vi "initUI.vi"(8 "Error In":errorcluster, 11 "UI Elements Cluster":T1) -> (0 "Error Out":errorcluster)   [LabVIEW 2018]
uses:
  controls/mainAppElementsCluster.ctl
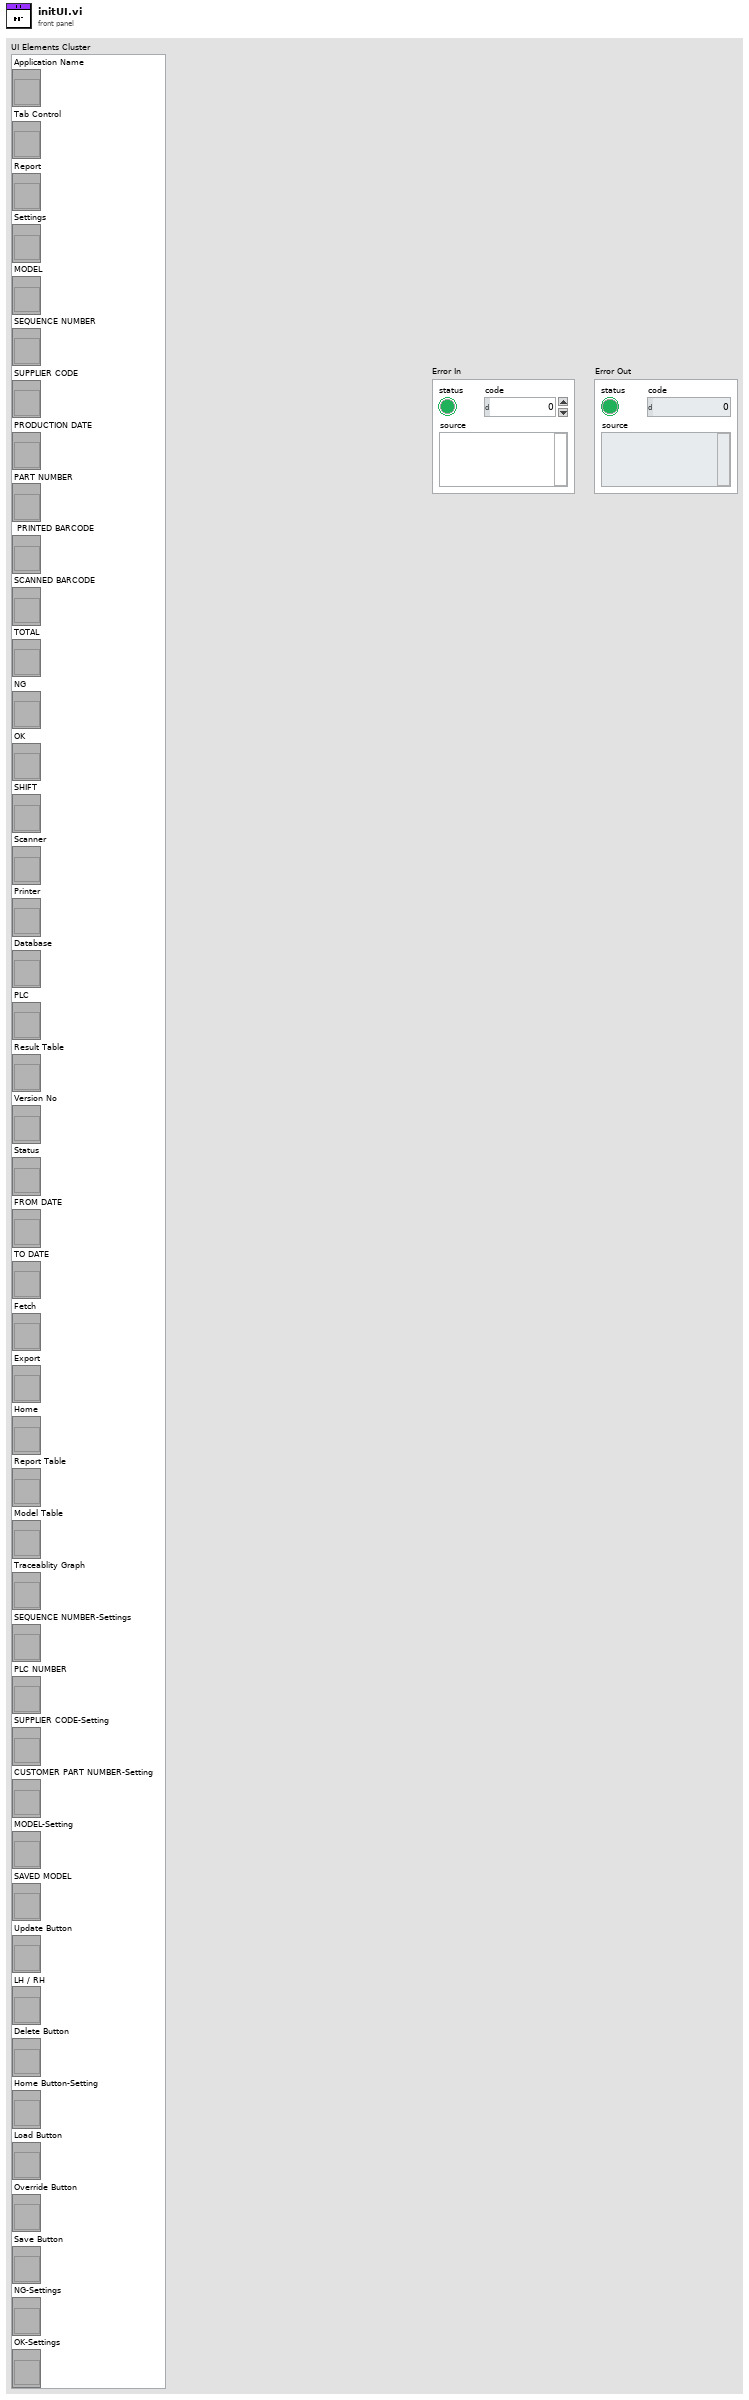
[diagram p1: front panel]
types:
  T1 = typedef "mainAppElementsCluster.ctl" = cluster{"Application Name":refnum<vi>, "Tab Control":refnum<vi>, "Status":refnum<vi>, "Version No":refnum<vi>, "Result Table":refnum<vi>, "PLC":refnum<vi>, "Database":refnum<vi>, "Printer":refnum<vi>, "Scanner":refnum<vi>, "SHIFT":refnum<vi>, "OK":refnum<vi>, "NG":refnum<vi>, "TOTAL":refnum<vi>, "SCANNED BARCODE":refnum<vi>, " PRINTED BARCODE":refnum<vi>, "PART NUMBER":refnum<vi>, "PRODUCTION DATE":refnum<vi>, "SUPPLIER CODE":refnum<vi>, "SEQUENCE NUMBER":refnum<vi>, "MODEL":refnum<vi>, "Settings":refnum<vi>, "Report":refnum<vi>, "Report Table":refnum<vi>, "Home":refnum<vi>, "Export":refnum<vi>, "Fetch":refnum<vi>, "TO DATE":refnum<vi>, "FROM DATE":refnum<vi>, "Model Table":refnum<vi>, "Traceablity Graph":refnum<vi>, "Override Button":refnum<vi>, "Load Button":refnum<vi>, "Home Button-Setting":refnum<vi>, "Delete Button":refnum<vi>, "Update Button":refnum<vi>, "Save Button":refnum<vi>, "SEQUENCE NUMBER-Settings":refnum<vi>, "PLC NUMBER":refnum<vi>, "LH / RH":refnum<vi>, "SUPPLIER CODE-Setting":refnum<vi>, "CUSTOMER PART NUMBER-Setting":refnum<vi>, "MODEL-Setting":refnum<vi>, "SAVED MODEL":refnum<vi>, "NG-Settings":refnum<vi>, "OK-Settings":refnum<vi>}
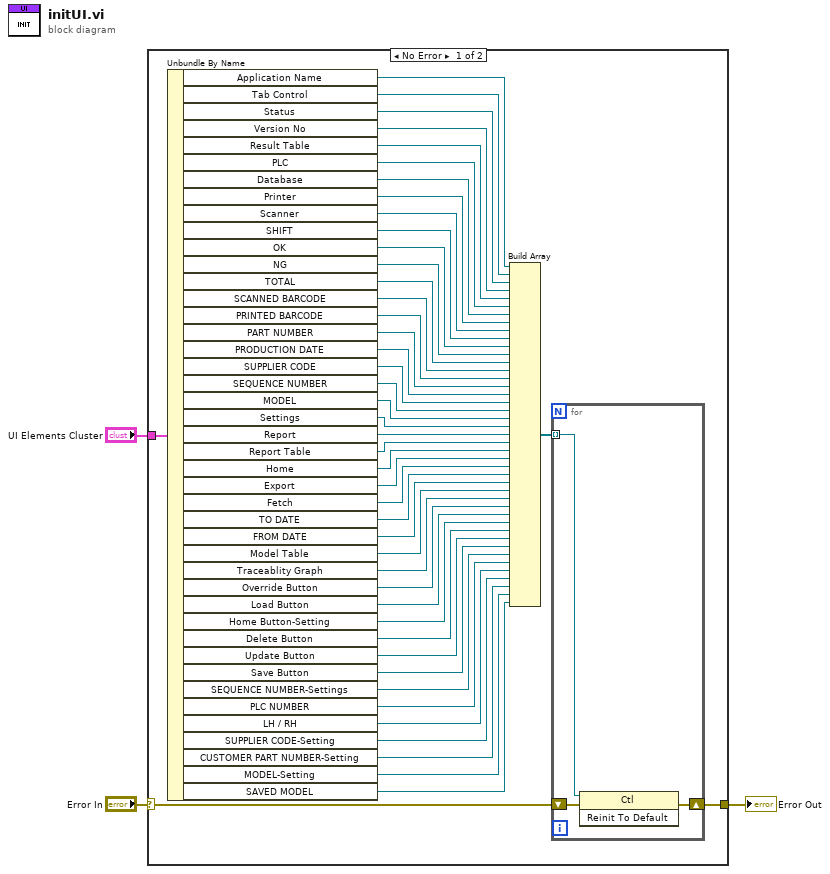
[diagram p0: block diagram]
diagram:
  n1 = case shown="No Error" "Error In" {
    selector: "Error In" -> [w12 w54]
    tunnel: [w13 w54] -> w2
    tunnel: "UI Elements Cluster" -> [w50 _]
    frame No Error {
      n2 = Unbundle By Name(w50) -> ("Application Name"=w11:refnum<vi>, "Tab Control"=w49:refnum<vi>, "Status"=w48:refnum<vi>, "Version No"=w47:refnum<vi>, "Result Table"=w46:refnum<vi>, "PLC"=w7:refnum<vi>, "Database"=w6:refnum<vi>, "Printer"=w5:refnum<vi>, "Scanner"=w4:refnum<vi>, "SHIFT"=w9:refnum<vi>, "OK"=w45:refnum<vi>, "NG"=w44:refnum<vi>, "TOTAL"=w43:refnum<vi>, "SCANNED BARCODE"=w42:refnum<vi>, "PRINTED BARCODE"=w41:refnum<vi>, "PART NUMBER"=w40:refnum<vi>, "PRODUCTION DATE"=w10:refnum<vi>, "SUPPLIER CODE"=w39:refnum<vi>, "SEQUENCE NUMBER"=w38:refnum<vi>, "MODEL"=w8:refnum<vi>, "Settings"=w37:refnum<vi>, "Report"=w36:refnum<vi>, "Report Table"=w35:refnum<vi>, "Home"=w34:refnum<vi>, "Export"=w33:refnum<vi>, "Fetch"=w32:refnum<vi>, "TO DATE"=w31:refnum<vi>, "FROM DATE"=w30:refnum<vi>, "Model Table"=w29:refnum<vi>, "Traceablity Graph"=w28:refnum<vi>, "Override Button"=w27:refnum<vi>, "Load Button"=w26:refnum<vi>, "Home Button-Setting"=w25:refnum<vi>, "Delete Button"=w24:refnum<vi>, "Update Button"=w23:refnum<vi>, "Save Button"=w22:refnum<vi>, "SEQUENCE NUMBER-Settings"=w21:refnum<vi>, "PLC NUMBER"=w20:refnum<vi>, "LH / RH"=w19:refnum<vi>, "SUPPLIER CODE-Setting"=w18:refnum<vi>, "CUSTOMER PART NUMBER-Setting"=w17:refnum<vi>, "MODEL-Setting"=w16:refnum<vi>, "SAVED MODEL"=w15:refnum<vi>)
      n3 = Build Array(w11, w49, w48, w47, w46, w7, w6, w5, w4, w9, w45, w44, w43, w42, w41, w40, w10, w39, w38, w8, w37, w36, w35, w34, w33, w32, w31, w30, w29, w28, w27, w26, w25, w24, w23, w22, w21, w20, w19, w18, w17, w16, w15) -> (w14:refnum<vi>[])
      n4 = for {
        tunnel: w14 -> [w53] mode=indexing
        shift-right: [w51] -> w13
        shift-left: w12 -> [w52]
        n5 = invoke class="Ctl" method="Reinit To Default"(reference=w53, error in=w52) -> (error out=w51:errorcluster)  [unwired: 1 in, 2 out]
      }
    }
    frame Error {
    }
  }
  "Error Out" <- w2
